vi "setUp.vi"(8 "error in (no error)":errorcluster, 11 "reference in":refnum<class "csm-ini-variable-addon.lvclass">) -> (0 "error out":errorcluster, 3 "reference out":refnum<class "csm-ini-variable-addon.lvclass">)   [LabVIEW 2017, in "csm-ini-variable-addon.lvclass"]
doc: "setUp runs prior to the test method during test execution. Use this method to initialize any object data required by your tests."
uses:
  csm-ini-variable-addon.lvclass
  C:/Program Files (x86)/National Instruments/LabVIEW 2017/vi.lib/addons/_JKI Toolkits/VI Tester/TestCase.llb/TestCase.lvclass
  csm-ini-variable-addon.lvclass/csm-ini-variable-addon.ctl
  <vilib>/addons/_JKI Toolkits/VI Tester/TestCase.llb/TestCase.lvclass
  INI-Static-Variable-Support/INI-Static-Variable-Support.lvlib
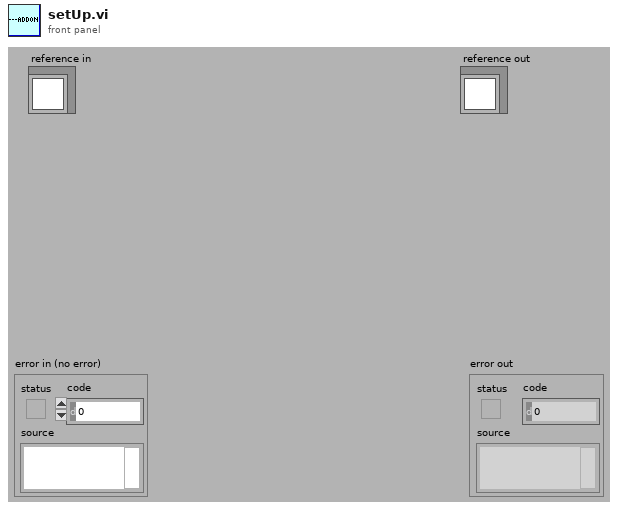
[diagram p1: front panel]
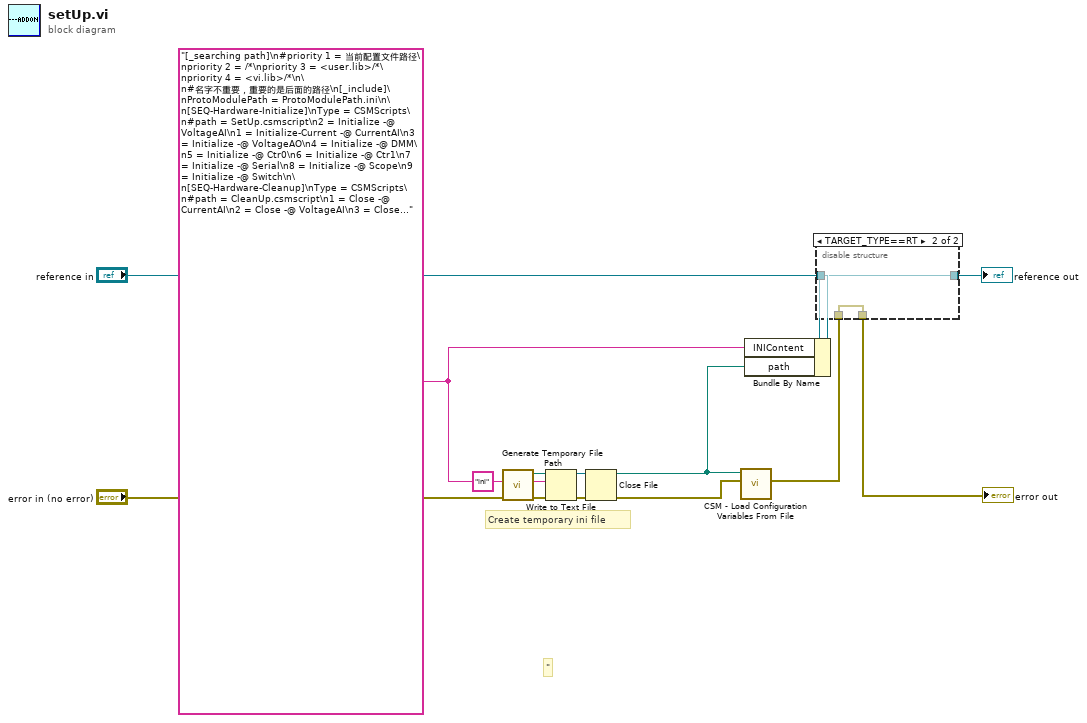
[diagram p0: block diagram]
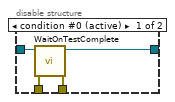
[diagram p2: hidden frame]
diagram:
  w1 = "[_searching path]\n#priority 1 = 当前配置文件路径\npriority 2 = /*\npriority 3 = <user.lib>/*\npriority 4 = <vi.lib>/*\n\n#名字不重要，重要的是后面的路径\n[_include]\nProtoModulePath = ProtoModulePath.ini\n\n[SEQ-Hardware-Initialize]\nType = CSMScripts\n#path = SetUp.csmscript\n2 = Initialize -@ VoltageAI\n1 = Initialize-Current -@ CurrentAI\n3 = Initialize -@ VoltageAO\n4 = Initialize -@ DMM\n5 = Initialize -@ Ctr0\n6 = Initialize -@ Ctr1\n7 = Initialize -@ Serial\n8 = Initialize -@ Scope\n9 = Initialize -@ Switch\n\n[SEQ-Hardware-Cleanup]\nType = CSMScripts\n#path = CleanUp.csmscript\n1 = Close -@ CurrentAI\n2 = Close -@ VoltageAI\n3 = Close -@ VoltageAO\n4 = Close -@ DMM\n5 = Close -@ Ctr0\n6 = Close -@ Ctr1\n7 = Close -@ Serial\n8 = Close -@ Scope\n9 = Close -@ Switch\n\n[bug]\nvaluewithbackslash = \\10folder\nvaluewithbackslash2 = \"\\10folder\""
  # "\""
  # "Create temporary ini file"
  n1 = call <vilib>:"Generate Temporary File Path.vi"("error in (no error)"="error in (no error)", "Temporary File Extension (tmp)"="ini") -> ("error out"=w10:errorcluster, "Unique Temporary File Path"=w7:path)  [unwired: 8 in]
  n2 = Write to Text File(file (use dialog)=w7, text=w1, error in=w10) -> (refnum out=w6:refnum<file>, error out=w8:errorcluster)  [unwired: 1 in, 1 out]
  n3 = Close File(refnum=w6, error in=w8) -> (path=w4:path, error out=w3:errorcluster)
  n4 = call "CSM - Load Configuration Variables From File.vi"("error in (no error)"=w3, "Path"=w4) -> ("error out"=w2:errorcluster)  [unwired: 7 in]
  n5 = Bundle By Name(cluster="reference in", "INIContent"=w1, "path"=w4) -> (w11:refnum<class "csm-ini-variable-addon.lvclass">)
  n6 = disable-structure "Conditional Disable Structure" shown="TARGET_TYPE==RT" {
    disable-tunnel: w2 -> [w18 w19]
    disable-tunnel: [w17 w19] -> w14
    disable-tunnel: [w16 w20] -> w12
    disable-tunnel: w11 -> [w15 w20]
    frame condition #0 (active) {
      n7 = call <vilib>:"WaitOnTestComplete.vi"("error in (no error)"=w18, "TestCase in"=w15) -> ("error out"=w17:errorcluster, "TestCase out"=w16:refnum<class "csm-ini-variable-addon.lvclass">)  [unwired: 8 in]
    }
    frame condition #1 {
    }
  }
  "error out" <- w14
  "reference out" <- w12
